vi "ConvolveFile.vi"(11 "Old Files":T1[](array[typedef])) -> ()   [LabVIEW 2022 SP3]
uses:
  Curtin1_Label.ctl
panel:
  in  "Right channel":u16(ring) items=["JacksonStrad H.AvC", "Titian Strad H.AvC", "Titian Strad H.AvC", "Titian Strad V.AvC"]
  out "ratio":dbl format="%0.2e"
  in  "Musical Piece":enum32{"Default", "Advanced"}(tab)
  in  "Path":path
  in  "save":bool
  in  "Sampling rate":u16=48000
  out "FRF":cluster{"t0":dbl, "dt":dbl, dbl[]}[](graph)=[{"t0"=0.0, "dt"=0.732421875, array[13995 elements]}, {"t0"=0.0, "dt"=0.732421875, array[13995 elements]}]
  out "PointIdx":i32=359
  out "CursLoc":cluster{"X":dbl, "Y":dbl}={"X"=262.939453125, "Y"=26.045098132964196}
  out "CursIdx":i32=1
  in  "Play 2":bool
  in  "Play":bool
  in  "Save Convolve":bool
  in  "Left channel":u16(ring) items=["JacksonStrad H.AvC", "Titian Strad H.AvC", "Titian Strad H.AvC", "Titian Strad V.AvC"]
  # "Tchaikovsky Violin Concerto"
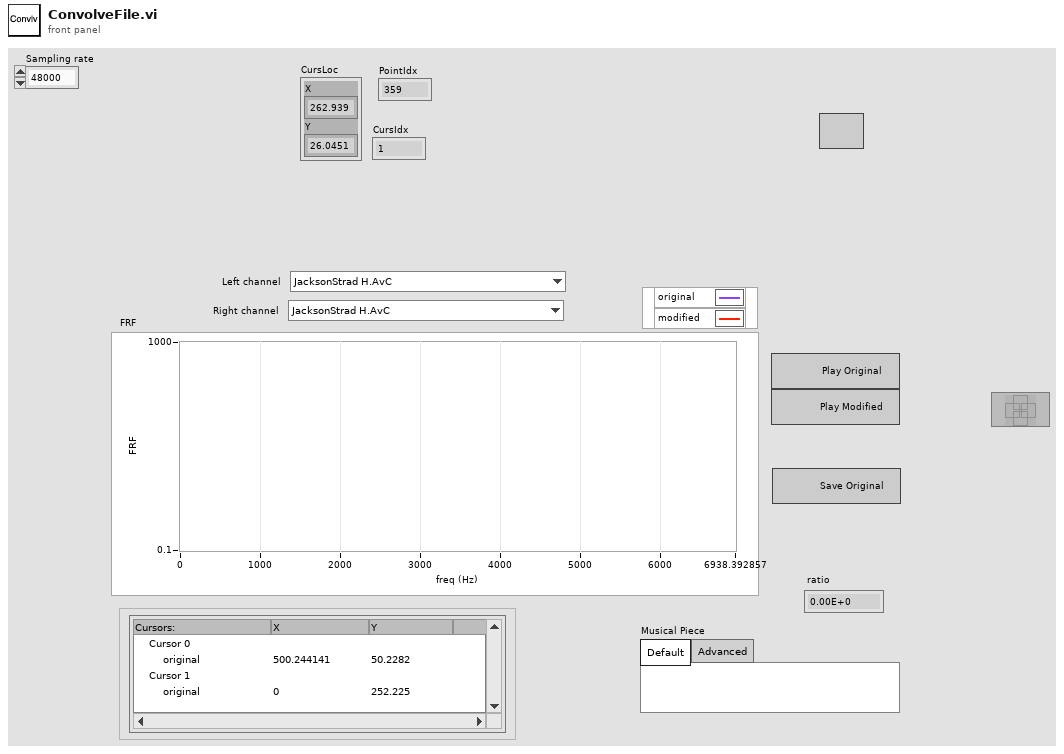
[diagram p1: front panel]
types:
  T1 = typedef "Curtin1_Label.ctl" = cluster{"Show?":bool, "Name":string, "Color":u32, "Path":path, "Show Notes":bool, "correlate":bool}
  T2 = typedef "PreferencesControl.ctl" = cluster{"Name of test":string, "Date":timestamp, "Location":string, "Template":string, "Soundcard":string, "resolution":u16, "Sampling rate":u16, "Ch1 Gain ":dbl, "Ch2 Gain":dbl, "Sample time (s)":dbl, "Pre-trigger (s)":dbl, "Hammer Threshold":dbl, "Positions":i16, "Taps/Position":i16, "Set Names":string, "Freq resolution":dbl, "Hammer cutoff":dbl, "Mic cutoff":dbl, "Double bounce ":dbl, "Hammer Cal":dbl, "dB Offset":dbl, "Accel Cal":dbl, "Vibrometer Cal":dbl, "Mic Cal":dbl, "Output":u16, "Voltage Cal":dbl, "Vibrometer Port":refnum<visa-resource-name>, "Range":u16, "High Pass":u16, "Bandwidth":u16, "X Range":cluster{"Minimum":dbl, "Maximum":dbl, "Increment":dbl, "Minor Increment":dbl, "Start":dbl}[], "Y Range":cluster{"Minimum":dbl, "Maximum":dbl, "Increment":dbl, "Minor Increment":dbl, "Start":dbl}[], "dB Spread":dbl, "Trigger":u16, "Ch_1":u8, "Ch_2":u8, "flip?":bool, "60Hz":bool, "Time offset":dbl, "Piezo Cal":dbl, "Default Notes":string, "Tom":bool}
  T3 = typedef "LVCursorListTypeDef.ctl" = cluster{"Name":string, "Color":u32, "Style":u8, "Point Style":u8, "Name Visible":bool, "Allow Drag":bool, "Cursor Mode":u32, "Plot":i32, "Index":i32, "Position":cluster{"X":dbl, "Y":dbl}, "X Scale":u32, "Y Scale":u32, "Watch Plots":i32[], "Watch All Plots":bool, "Plot Area":i32, "Label Offset":cluster{"X":dbl, "Y":dbl}}[]
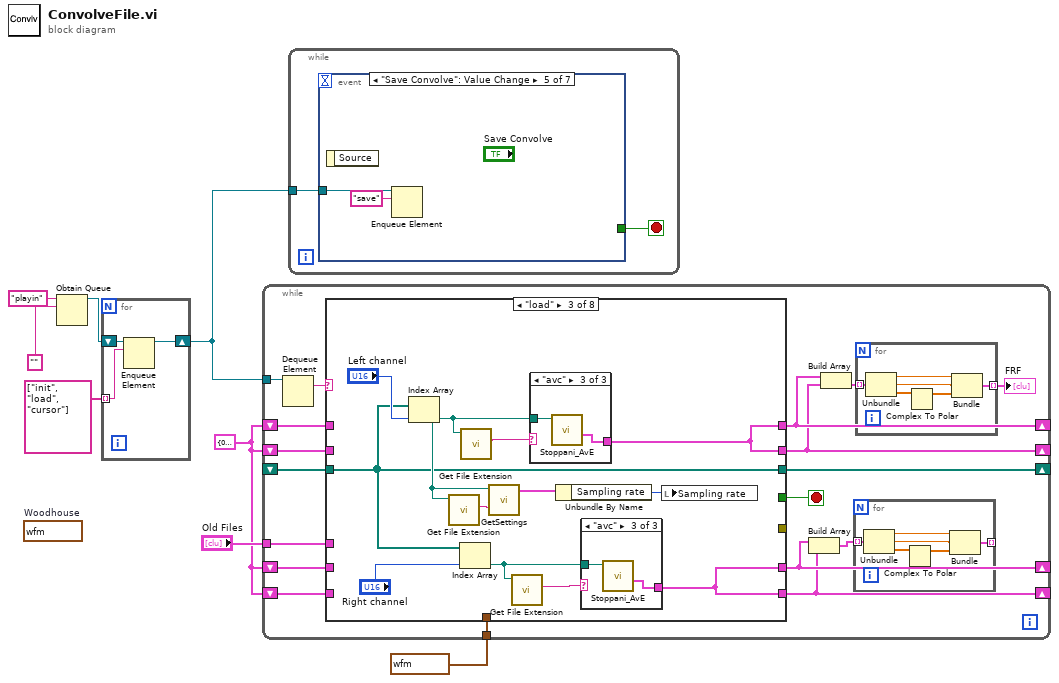
[diagram p0: block diagram]
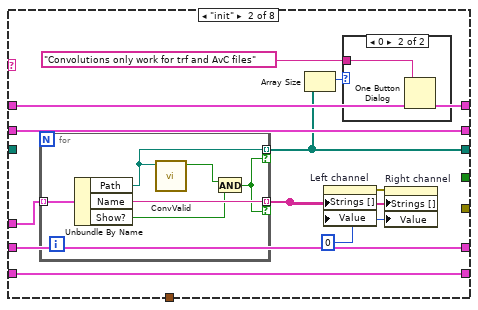
[diagram p3: hidden frame]
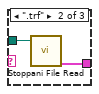
[diagram p6: hidden frame]
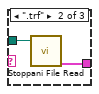
[diagram p8: hidden frame]
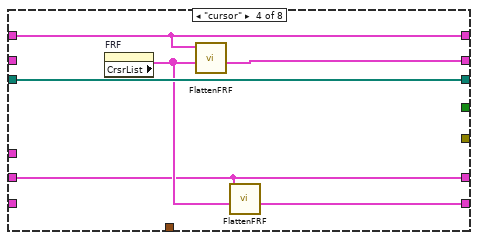
[diagram p9: hidden frame]
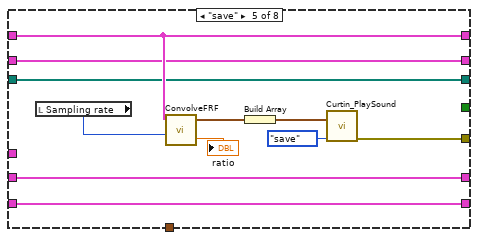
[diagram p10: hidden frame]
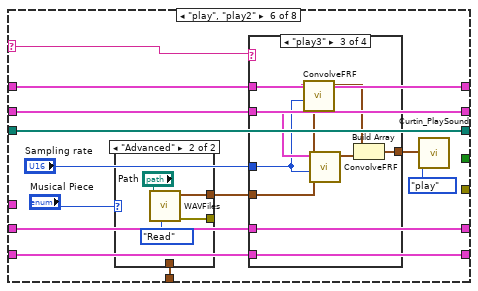
[diagram p11: hidden frame]
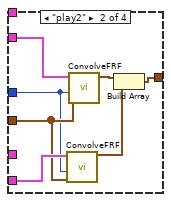
[diagram p13: hidden frame]
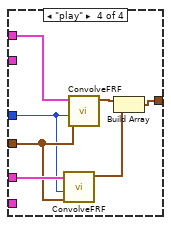
[diagram p14: hidden frame]
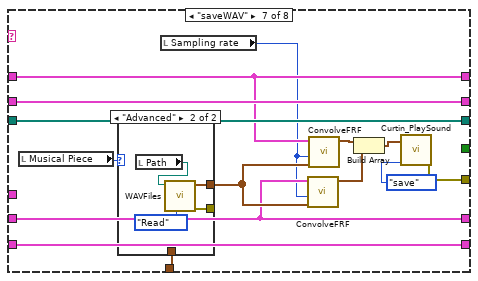
[diagram p16: hidden frame]
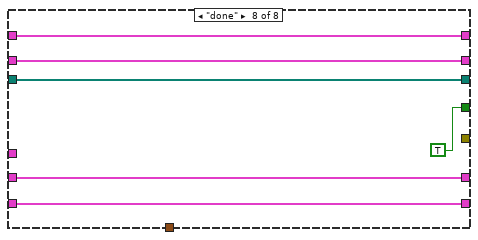
[diagram p18: hidden frame]
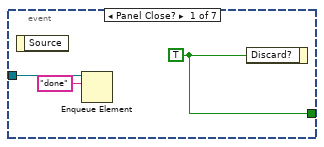
[diagram p19: hidden frame]
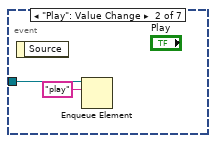
[diagram p20: hidden frame]
diagram:
  (unwired) waveform(dbl)[] [{"t0"=timestamp(0 s since 1904-01-01), "dt"=2.5e-05, "Y"=array[400000 elements]}]  # Woodhouse
  w2 = cluster{"t0":dbl, "dt":dbl, "Y":cdb[]} {"t0"=0.0, "dt"=0.0, "Y"=[]} ("Complex FRF")
  n1 = Obtain Queue(name (unnamed)="playin", element data type="" ("element")) -> (queue out=w8:refnum<queue>)  [unwired: 3 in, 2 out]
  n2 = for {
    shift-right: [w10] -> w7
    shift-left: w8 -> [w11]
    tunnel: string[] ["init", "load", "cursor"] -> [w9] mode=indexing
    n3 = Enqueue Element(queue=w11, element=w9) -> (queue out=w10:refnum<queue>)  [unwired: 2 in, 2 out]
  }
  n4 = while {
    tunnel: w7 -> [w29]
    shift-right: [w23] -> _
    shift-left: w2 -> [w26]
    shift-right: [w22] -> _
    shift-left: w2 -> [w25]
    tunnel: "Old Files" -> [w20]
    shift-right: [w19] -> _
    shift-left: _ -> [w18]
    shift-right: [w16] -> _
    shift-left: w2 -> [w14]
    shift-right: [w15] -> _
    shift-left: w2 -> [w13]
    tunnel: waveform(dbl)[] [{"t0"=timestamp(0 s since 1904-01-01), "dt"=2.0833333333333333e-05, "Y"=array[288010 elements]}, {"t0"=timestamp(0 s since 1904-01-01), "dt"=2.0833333333333333e-05, "Y"=array[288010 elements]}] ("musical piece") -> [w12]
    stop <- w27 stop-if-true
    n5 = Dequeue Element(queue=w29) -> (element=w28:string)  [unwired: 2 in, 3 out]
    n6 = case shown="\"load\"" w28 {
      selector: w28 -> [_ _ _ _ _ w107 _ _]
      tunnel: [_ _ _ _ _ _ _ TRUE] -> w27
      tunnel: [w46 w57 w76 w89 w100 w106 w149 w163] -> w23
      tunnel: w26 -> [w46 w57 _ w89 w100 w106 w149 w163]
      tunnel: w25 -> [w45 w56 _ _ w98 w111 w152 w162]
      tunnel: [w45 w56 w76 w88 w98 w111 w152 w162] -> w22
      tunnel: w20 -> [_ w55 _ _ _ _ _ _]
      tunnel: [w44 w54 w67 w90 w97 w110 w151 w161] -> w19
      tunnel: w18 -> [w44 _ w67 w90 w97 w110 w151 w161]
      tunnel: [w43 w48 w65 w86 w93 w105 w148 w160] -> w16
      tunnel: [w42 w47 w65 w85 w92 w104 w147 w159] -> w15
      tunnel: w14 -> [w43 w48 _ w86 w93 w105 w148 w160]
      tunnel: w13 -> [w42 w47 _ _ w92 w104 w147 w159]
      tunnel: w12 -> [_ _ _ _ _ w102 w141 _]
      tunnel: [_ _ _ _ w91 _ w140 _] -> _
      frame Default {
      }
      frame "init" {
        w49 = 0
        n7 = for {
          tunnel: [w64] -> w50 mode=indexing if=w60
          tunnel: [w62] -> w54 mode=indexing if=w60
          tunnel: w55 -> [w63] mode=indexing
          n8 = Unbundle By Name(w63) -> ("Path"=w62:path, "Name"=w64:string, "Show?"=w61:bool)
          n9 = call "ConvValid.vi"("Path"=w62) -> ("Valid"=w59:bool)  [unwired: 10 in]
          n10 = And(x=w59, y=w61) -> (x .and. y?=w60:bool)
        }
        n11 = Array Size(array=w54) -> (size(s)=w53:i32)
        n12 = property on="Left channel" class="Ring (strict)"("Strings []"=w50, "Value"=w49) -> (error out=w51:errorcluster)  [unwired: 2 in, 1 out]
        n13 = case shown="0" w53 {
          tunnel: "Convolutions only work for trf and AvC files" ("element") -> [_ w58]
          frame Default {
          }
          frame 0 {
            n14 = One Button Dialog(message=w58) -> ()  [unwired: 1 in, 1 out]
          }
        }
        n15 = property on="Right channel" class="Ring (strict)"(error in=w51, "Strings []"=w50, "Value"=w49) -> ()  [unwired: 1 in, 2 out]
      }
      frame "load" {
        n16 = Index Array(array=w67, index="Left channel") -> (element=w71:path)
        n17 = call <vilib>:"Get File Extension.vi"("file"=w71) -> ("lowercase file extension"=w75:string)  [unwired: 6 in, 4 out]
        n18 = Index Array(array=w67, index="Right channel") -> (element=w68:path)
        n19 = call <vilib>:"Get File Extension.vi"("file"=w71) -> ("lowercase file extension"=w70:string)  [unwired: 6 in, 4 out]
        n20 = call "GetSettings.vi"("lowercase file extension"=w75, "wavform file"=w71) -> ("Settings"=w74:T2)  [unwired: 8 in, 1 out]
        n21 = call <vilib>:"Get File Extension.vi"("file"=w68) -> ("lowercase file extension"=w69:string)  [unwired: 6 in, 4 out]
        n22 = case shown="\"avc\"" w70 {
          tunnel: [_ w82 w83] -> w76
          tunnel: w71 -> [_ w81 w84]
          frame Default {
          }
          frame ".trf" {
            n23 = call "Stoppani File Read.vi"("String in"=w81) -> ("Complex FRF"=w82:cluster{"t0":dbl, "dt":dbl, "Y":cdb[]})  [unwired: 2 in, 3 out]
          }
          frame "avc" {
            n24 = call "Stoppani_AvE.vi"("file (use dialog)"=w84) -> ("Complex FRF"=w83:cluster{"t0":dbl, "df":dbl, "Y":cdb[]})  [unwired: 7 in, 3 out]
          }
        }
        n25 = Unbundle By Name(w74) -> ("Sampling rate"=w73:u16)
        n26 = case shown="\"avc\"" w69 {
          tunnel: [_ w78 w79] -> w65
          tunnel: w68 -> [_ w77 w80]
          frame Default {
          }
          frame ".trf" {
            n27 = call "Stoppani File Read.vi"("String in"=w77) -> ("Complex FRF"=w78:cluster{"t0":dbl, "dt":dbl, "Y":cdb[]})  [unwired: 2 in, 3 out]
          }
          frame "avc" {
            n28 = call "Stoppani_AvE.vi"("file (use dialog)"=w80) -> ("Complex FRF"=w79:cluster{"t0":dbl, "df":dbl, "Y":cdb[]})  [unwired: 7 in, 3 out]
          }
        }
        n29 = local write "Sampling rate"(w73) -> ()
      }
      frame "cursor" {
        n30 = property on="FRF" class="WFGraph (strict)"() -> ("CrsrList"=w87:T3)  [unwired: 2 in, 2 out]
        n31 = call "FlattenFRF.vi"("CrsrList"=w87, "Data in"=w89) -> ("Data out"=w88:cluster{"t0":dbl, "dt":dbl, "Y":cdb[]})  [unwired: 9 in]
        n32 = call "FlattenFRF.vi"("CrsrList"=w87, "Data in"=w86) -> ("Data out"=w85:cluster{"t0":dbl, "dt":dbl, "Y":cdb[]})  [unwired: 9 in]
      }
      frame "save" {
        n33 = local read "Sampling rate"() -> (w96:u16)
        n34 = call "ConvolveFRF.vi"("Sampling rate"=w96, "Complex FRF"=w100) -> ("Convolution"=w99:waveform(dbl), "ratio"=→"ratio":dbl)  [unwired: 6 in, 2 out]
        n35 = Build Array(w99) -> (w101:waveform(dbl)[])
        n36 = call "Curtin_PlaySound.vi"("Task"=enum16{"play", "save"}."save", "all waveforms"=w101) -> ("error out"=w91:errorcluster)  [unwired: 9 in]
      }
      frame "play", "play2" {
        n37 = case shown="\"Advanced\"" "Musical Piece" {
          tunnel: [w135 w138] -> w109
          tunnel: [_ w136] -> _
          tunnel: w102 -> [w135 _]
          frame Default {
          }
          frame "Advanced" {
            n38 = call "WAVFiles.vi"("Task"=enum16{"Read", "Write", "wfm"}."Read", "WAV File"="Path") -> ("error out"=w136:errorcluster, "Data"=w138:waveform(dbl)[])  [unwired: 6 in, 2 out]
          }
        }
        n39 = case shown="\"play3\"" w107 {
          tunnel: [_ w120 w127 w134] -> w113
          tunnel: "Sampling rate" -> [_ w115 w123 w129]
          tunnel: w111 -> [_ w119 w126 _]
          tunnel: w109 -> [_ w116 w122 w130]
          tunnel: w106 -> [_ _ w124 w132]
          tunnel: w105 -> [_ _ _ w131]
          tunnel: w104 -> [_ w117 _ _]
          frame Default {
          }
          frame "play2" {
            n40 = call "ConvolveFRF.vi"("musical piece"=w116, "Sampling rate"=w115, "Complex FRF"=w117) -> ("Convolution"=w114:waveform(dbl))  [unwired: 5 in, 3 out]
            n41 = call "ConvolveFRF.vi"("musical piece"=w116, "Sampling rate"=w115, "Complex FRF"=w119) -> ("Convolution"=w118:waveform(dbl))  [unwired: 5 in, 3 out]
            n42 = Build Array(w118, w114) -> (w120:waveform(dbl)[])
          }
          frame "play3" {
            n43 = call "ConvolveFRF.vi"("musical piece"=w122, "Sampling rate"=w123, "Complex FRF"=w124) -> ("Convolution"=w121:waveform(dbl))  [unwired: 5 in, 3 out]
            n44 = call "ConvolveFRF.vi"("musical piece"=w122, "Sampling rate"=w123, "Complex FRF"=w126) -> ("Convolution"=w125:waveform(dbl))  [unwired: 5 in, 3 out]
            n45 = Build Array(w121, w125) -> (w127:waveform(dbl)[])
          }
          frame "play" {
            n46 = call "ConvolveFRF.vi"("musical piece"=w130, "Sampling rate"=w129, "Complex FRF"=w131) -> ("Convolution"=w128:waveform(dbl))  [unwired: 5 in, 3 out]
            n47 = call "ConvolveFRF.vi"("musical piece"=w130, "Sampling rate"=w129, "Complex FRF"=w132) -> ("Convolution"=w133:waveform(dbl))  [unwired: 5 in, 3 out]
            n48 = Build Array(w133, w128) -> (w134:waveform(dbl)[])
          }
        }
        n49 = call "Curtin_PlaySound.vi"("Task"=enum16{"play", "save"}."play", "all waveforms"=w113) -> ()  [unwired: 9 in, 1 out]
      }
      frame "saveWAV" {
        n50 = local read "Musical Piece"() -> (w142:enum32{"Default", "Advanced"})
        n51 = case shown="\"Advanced\"" w142 {
          tunnel: [w154 w157] -> w150
          tunnel: [_ w156] -> _
          tunnel: w141 -> [w154 _]
          frame Default {
          }
          frame "Advanced" {
            n52 = local read "Path"() -> (w155:path)
            n53 = call "WAVFiles.vi"("Task"=enum16{"Read", "Write", "wfm"}."Read", "WAV File"=w155) -> ("error out"=w156:errorcluster, "Data"=w157:waveform(dbl)[])  [unwired: 6 in, 2 out]
          }
        }
        n54 = local read "Sampling rate"() -> (w143:u16)
        n55 = call "ConvolveFRF.vi"("musical piece"=w150, "Sampling rate"=w143, "Complex FRF"=w148) -> ("Convolution"=w144:waveform(dbl))  [unwired: 5 in, 3 out]
        n56 = call "ConvolveFRF.vi"("musical piece"=w150, "Sampling rate"=w143, "Complex FRF"=w149) -> ("Convolution"=w145:waveform(dbl))  [unwired: 5 in, 3 out]
        n57 = Build Array(w145, w144) -> (w153:waveform(dbl)[])
        n58 = call "Curtin_PlaySound.vi"("Task"=enum16{"play", "save"}."save", "all waveforms"=w153) -> ("error out"=w140:errorcluster)  [unwired: 9 in]
      }
      frame "done" {
      }
    }
    n59 = Build Array(w16, w15) -> (w17:cluster{"t0":dbl, "dt":dbl, "Y":cdb[]}[])
    n60 = Build Array(w23, w22) -> (w21:cluster{"t0":dbl, "dt":dbl, "Y":cdb[]}[])
    n61 = for {
      tunnel: [w33] -> _ mode=indexing
      tunnel: w17 -> [w30] mode=indexing
      n62 = Unbundle(w30) -> ("t0"=w35:dbl, "dt"=w34:dbl, "Y"=w31:cdb[])
      n63 = Complex To Polar(r * e^(i*theta)=w31) -> (r=w32:dbl[])  [unwired: 1 out]
      n64 = Bundle("t0"=w35, "dt"=w34, w32) -> (w33:cluster{"t0":dbl, "dt":dbl, dbl[]})  [unwired: 1 in]
    }
    n65 = for {
      tunnel: [w39] -> w24 mode=indexing
      tunnel: w21 -> [w36] mode=indexing
      n66 = Unbundle(w36) -> ("t0"=w41:dbl, "dt"=w40:dbl, "Y"=w37:cdb[])
      n67 = Complex To Polar(r * e^(i*theta)=w37) -> (r=w38:dbl[])  [unwired: 1 out]
      n68 = Bundle("t0"=w41, "dt"=w40, w38) -> (w39:cluster{"t0":dbl, "dt":dbl, dbl[]})  [unwired: 1 in]
    }
    "FRF" <- w24
  }
  n69 = while {
    tunnel: w7 -> [w166]
    stop <- w165 stop-if-true
    n70 = event shown="[4] \"Save Convolve\": Value Change" {
      selector: _ -> [_ _ _ _ _ _ _]
      dyn-events: _ -> [_ _ _ _ _ _ _]
      timeout: _ -> [_ _ _ _ _ _ _]
      tunnel: w166 -> [w169 w171 w173 w175 w177 w182 w186]
      tunnel: [w168 _ _ _ _ _ _] -> w165
      event Panel Close? {
        w168 = TRUE ("Discard?")
        n71 = event-data() -> ()  [unwired: 1 in, 1 out]
        n72 = Enqueue Element(queue=w169, element="done") -> ()  [unwired: 2 in, 3 out]
        n73 = event-data("Discard?"=w168) -> ()  [unwired: 1 in, 1 out]
      }
      event "Play": Value Change {
        n74 = event-data() -> ()  [unwired: 1 in, 1 out]
        n75 = Enqueue Element(queue=w171, element="play") -> ()  [unwired: 2 in, 3 out]
      }
      event "Play 2": Value Change {
        n76 = event-data() -> ()  [unwired: 1 in, 1 out]
        n77 = Enqueue Element(queue=w173, element="play2") -> ()  [unwired: 2 in, 3 out]
      }
      event "save": Value Change {
        n78 = event-data() -> ()  [unwired: 1 in, 1 out]
        n79 = Enqueue Element(queue=w175, element="saveWAV") -> ()  [unwired: 2 in, 3 out]
      }
      event "Save Convolve": Value Change {
        n80 = event-data() -> ()  [unwired: 1 in, 1 out]
        n81 = Enqueue Element(queue=w177, element="save") -> ()  [unwired: 2 in, 3 out]
      }
      event "FRF": Cursor Move {
        n82 = event-data() -> ("CursIdx"=→"CursIdx":i32, "PointIdx"=→"PointIdx":i32, "CursLoc"=→"CursLoc":cluster{"X":dbl, "Y":dbl})  [unwired: 1 in]
        n83 = Enqueue Element(queue=w182, element="cursor") -> ()  [unwired: 2 in, 3 out]
      }
      event "Left channel": Value Change {
        n84 = event-data() -> ()  [unwired: 1 in, 1 out]
        n85 = Enqueue Element(queue=w186, element="load") -> (queue out=w183:refnum<queue>)  [unwired: 2 in, 2 out]
        n86 = Enqueue Element(queue=w183, element="cursor") -> ()  [unwired: 2 in, 3 out]
      }
    }
  }
